vi "CRYInsert Custom Data.vi"(5 "sAction":string, 7 "Setup in":T6={"No.VI"=0, "Category"="", "StepName"="", "Seq setup flattened"="", "Comment"="", "Steps config."=[], "Jump config"=[], "Start"=0.0, "Increment"=0.0, "Name"="Pa", "Unit"="Pa", "Y data"=1, "Y prefix"="", "Y dB ref"=1.0, "Y unit"="", "Repeat State Array"=[]} {"Repeat State Array"."Start" format="%#_5g"; "Y dB ref" format="%.1f"; "Y data" items=["dB", "Lin"]; "Start" format="%#_5g"}, 8 "Wave":T3[](array[typedef]) {"Y dB ref" format="%.1f"; "Y axis" items=["Log", "Lin"]; "Y data" items=["dB", "Lin"]; "X data" items=["dB", "Lin"]}, 9 "Results":T4 {"Margin" format="%.2f"}, 10 "Values":T1 {"Z data" items=["dB", "Lin"]; "X data" items=["dB", "Lin"]; "Y data" items=["dB", "Lin"]; "Z dB ref" format="%.1f"; "Z axis" items=["Log", "Lin"]; "X dB ref" format="%.1f"; "X axis" items=["Log", "Lin"]; "Y axis" items=["Log", "Lin"]; "Y dB ref" format="%.1f"; "Curve"."z" format="%.2f"; "Curve"."y" format="%.2f"; "Curve"."x" format="%.2f"}, 11 "Curves":T1 {"Z data" items=["dB", "Lin"]; "X data" items=["dB", "Lin"]; "Y data" items=["dB", "Lin"]; "Z dB ref" format="%.1f"; "Z axis" items=["Log", "Lin"]; "X dB ref" format="%.1f"; "X axis" items=["Log", "Lin"]; "Y axis" items=["Log", "Lin"]; "Y dB ref" format="%.1f"; "Curve"."z" format="%.2f"; "Curve"."y" format="%.2f"; "Curve"."x" format="%.2f"}) -> (2 "Inserted Names Out":string[](array[string]), 3 "Types Out":string[](array[string]))   [LabVIEW 2013]
uses:
  Typedef Control/CRYStep.ctl
  Typedef Control/CRYData Cluster Array.ctl
  Typedef Control/CRYData Cluster.ctl
  Typedef Control/CRYResult Cluster Array.ctl
  Typedef Control/CRYResult Cluster.ctl
  Typedef Control/CRYWaveform Cluster.ctl
  Task Sequence/CRYProject Run Control Global.vi
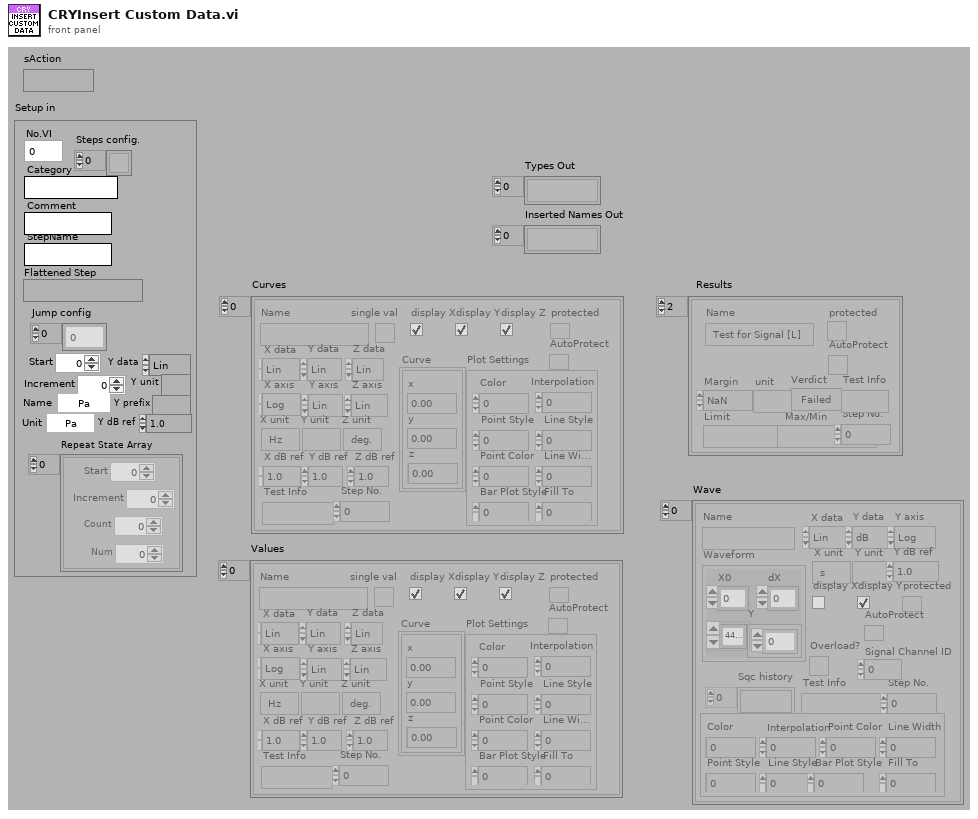
[diagram p1: front panel]
types:
  T1 = typedef "CRYData Cluster Array.ctl" = T2[]
  T2 = typedef "CRYData Cluster.ctl" = cluster{"Name":string, "Curve":cluster{"x":dbl, "y":dbl, "z":dbl}[], "X data":u16, "Y data":u16, "Z data":u16, "X axis":u16, "Y axis":u16, "Z axis":u16, "X unit":string, "Y unit":string, "Z unit":string, "X dB ref":dbl, "Y dB ref":dbl, "Z dB ref":dbl, "single val":bool, "protected":bool, "display X":bool, "display Y":bool, "display Z":bool, "Test Info":string, "Step No.":i32, "Plot Settings":cluster{"Color":u32, "Interpolation":u8, "Point Style":u8, "Line Style":u8, "Point Color":u32, "Line Width":u8, "Bar Plot Style":u8, "Fill To":i16}, "AutoProtect":bool}
  T3 = typedef "CRYWaveform Cluster.ctl" = cluster{"Waveform":cluster{"X0":dbl, "dX":dbl, "Y":sgl[]}, "X data":u16, "Y data":u16, "Y axis":u16, "X unit":string, "Y unit":string, "Y dB ref":dbl, "display Y":bool, "display X":bool, "Overload?":bool, "Test Info":string, "Step No.":i32, "Name":string, "protected":bool, "Sqc history":string[], "Signal Channel ID":i32, "Plot Settings":cluster{"Color":u32, "Interpolation":u8, "Point Style":u8, "Line Style":u8, "Point Color":u32, "Line Width":u8, "Bar Plot Style":u8, "Fill To":i16}, "AutoProtect":bool}
  T4 = typedef "CRYResult Cluster Array.ctl" = T5[]
  T5 = typedef "CRYResult Cluster.ctl" = cluster{"Name":string, "Margin":dbl, "unit":string, "Verdict":bool, "Limit":string, "Max/Min":string, "protected":bool, "Step No.":i32, "Test Info":string, "AutoProtect":bool}
  T6 = typedef "CRYStep.ctl" = cluster{"No.VI":i32, "Category":string, "StepName":string, "Seq setup flattened":string, "Comment":string, "Steps config.":bool[], "Jump config":i32[], "Start":dbl, "Increment":dbl, "Name":string, "Unit":string, "Y data":u16, "Y prefix":string, "Y dB ref":dbl, "Y unit":string, "Repeat State Array":cluster{"Start":dbl, "Increment":dbl, "Count":i32, "Num":i32}[]}
  T7 = cluster{"Start":dbl, "Increment":dbl, "Count":i32, "Num":i32}[]
  T8 = typedef "CRYWaveform Cluster Array.ctl" = T3[]
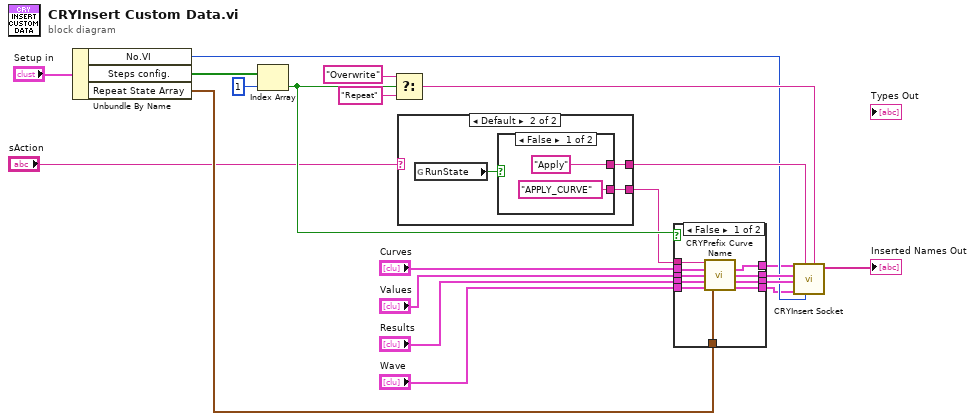
[diagram p0: block diagram]
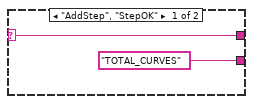
[diagram p2: hidden frame]
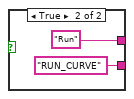
[diagram p3: hidden frame]
diagram:
  n1 = Unbundle By Name("Setup in") -> ("No.VI"=w10:i32, "Steps config."=w9:bool[], "Repeat State Array"=w8:T7)
  n2 = Index Array(array=w9, index=1) -> (element=w15:bool)
  n3 = Select(t="Overwrite" ("Y unit"), s=w15, f="Repeat") -> (s? t:f=w18:string)
  n4 = case shown="Default" "sAction" {
    selector: "sAction" -> [w23 _]
    tunnel: ["TOTAL_CURVES" ("Type In") w25] -> w13
    tunnel: [w23 w24] -> w12
    frame "AddStep", "StepOK" {
    }
    frame Default {
      n5 = global read "CRYProject Run Control Global.vi" "RunState"() -> (w26:bool)
      n6 = case shown="False" w26 {
        tunnel: ["Apply" ("sOption1") "Run" ("Type In")] -> w24
        tunnel: ["APPLY_CURVE" ("Type In") "RUN_CURVE" ("Type In")] -> w25
        frame False {
        }
        frame True {
        }
      }
    }
  }
  n7 = case shown="False" w15 {
    tunnel: "Values" -> [w40 w44]
    tunnel: "Results" -> [w39 w43]
    tunnel: [w38 w44] -> w17
    tunnel: [w37 w43] -> w16
    tunnel: w8 -> [w36 _]
    tunnel: w13 -> [w35 _]
    tunnel: "Curves" -> [w34 w42]
    tunnel: "Wave" -> [w33 w41]
    tunnel: [w32 w42] -> w2
    tunnel: [w31 w41] -> w1
    frame False {
      n8 = call "CRYPrefix Curve Name.vi"("Type In"=w35, "Curves In"=w34, "Values In"=w40, "Results In"=w39, "Waves In"=w33, "Repeat State Array In"=w36) -> ("Curves Out"=w32:T1, "Values Out"=w38:T1, "Results Out"=w37:T4, "Waves Out"=w31:T8)  [unwired: 6 in]
    }
    frame True {
    }
  }
  n9 = call "CRYInsert Socket.vi"("sOption2"=w18, "Step No."=w10, "sOption1"=w12, "Waves"=w1, "Results"=w16, "Values"=w17, "Curves"=w2) -> ("Inserted Names Out"=→"Inserted Names Out":string[])  [unwired: 4 in]
